vi "Enum Paths.vi"(8 "error in (no error)":errorcluster, 10 "Enum Type Name":string, 11 "LV-Protoc in":refnum<class "LV-Protoc.lvclass">) -> (0 "error out":errorcluster, 2 "Enum Paths":T1, 3 "LV-Protoc out":refnum<class "LV-Protoc.lvclass">)   [LabVIEW 2020, in "LV-Protoc.lvlib" / "LV-Protoc.lvclass"]
uses:
  LV-Protoc.lvclass
  Enumeration Paths.ctl
  LV-Protoc.lvclass/LV-Protoc.ctl
  LV-Protoc.lvlib
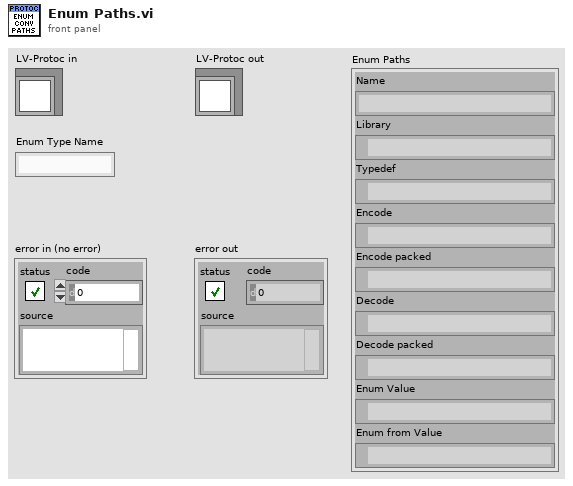
[diagram p1: front panel]
types:
  T1 = typedef "LV-Protoc.lvlib/Enumeration Paths.ctl" = cluster{"Name":string, "Library":path, "Typedef":path, "Encode":path, "Encode packed":path, "Decode":path, "Decode packed":path, "Enum Value":path, "Enum from Value":path}
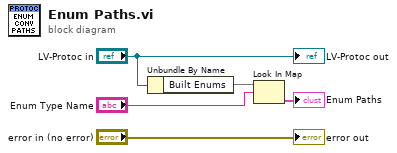
[diagram p0: block diagram]
diagram:
  n1 = Unbundle By Name("LV-Protoc in") -> ("Built Enums"=w5:map{string, T1})
  n2 = Look In Map(map=w5, key="Enum Type Name") -> (value=→"Enum Paths":T1)  [unwired: 1 in, 1 out]
  "error out" <- "error in (no error)"
  "LV-Protoc out" <- "LV-Protoc in"
